vi "Autonomous Independent.vi"() -> ()   [LabVIEW 2016]
doc: "This VI is called when autonomous begins, and will automatically be terminated when autonomous ends. You can carry out timed or sensor driven robot movement independently without needing to return to the caller."
uses:
  <vilib>/Rock Robotics/Network Tables/NT Read Number.vi
  <vilib>/Rock Robotics/WPI/Solenoid/WPI_SolenoidValue.ctl
panel:
  in  "Value":T1=enum."Forward"
  out "Auto Mode":dbl=3.0
  in  "Auton_Modes":T2(array[cluster])=[{"Actions"=[{"Effort"=0.55, "Duration"=3.5, "Action"=enum."Nothing"}, {"Effort"=0.0, "Duration"=0.0, "Action"=enum."Nothing"}]}, {"Actions"=[{"Effort"=0.0, "Duration"=1.0, "Action"=enum."Nothing"}, {"Effort"=0.75, "Duration"=5.0, "Action"=enum."Nothing"}, {"Effort"=0.0, "Duration"=1.0, "Action"=enum."Nothing"}]}, {"Actions"=[{"Effort"=1.0, "Duration"=3.0, "Action"=enum."Nothing"}, {"Effort"=0.0, "Duration"=1.0, "Action"=enum."Nothing"}, {"Effort"=0.75, "Duration"=3.5, "Action"=enum."Nothing"}, {"Effort"=0.0, "Duration"=1.0, "Action"=enum."Nothing"}]}, {"Actions"=[{"Effort"=0.0, "Duration"=0.5, "Action"=enum."Nothing"}, {"Effort"=0.8, "Duration"=5.28, "Action"=enum."Nothing"}, {"Effort"=0.0, "Duration"=1.0, "Action"=enum."Nothing"}, {"Effort"=-0.8, "Duration"=1.8, "Action"=enum."Nothing"}, {"Effort"=0.0, "Duration"=0.1, "Action"=enum."Nothing"}, {"Effort"=0.8, "Duration"=1.75, "Action"=enum."Nothing"}, {"Effort"=0.0, "Duration"=0.5, "Action"=enum."Nothing"}, {"Effort"=0.0, "Duration"=4.0, "Action"=enum."Nothing"}]}, {"Actions"=[{"Effort"=0.0, "Duration"=0.0, "Action"=enum."Nothing"}, {"Effort"=1.0, "Duration"=0.1, "Action"=enum."Nothing"}, {"Effort"=0.0, "Duration"=0.1, "Action"=enum."Nothing"}, {"Effort"=1.0, "Duration"=3.0, "Action"=enum."Nothing"}]}, {"Actions"=[{"Effort"=0.0, "Duration"=0.0, "Action"=enum."Nothing"}, {"Effort"=1.0, "Duration"=0.1, "Action"=enum."Nothing"}, {"Effort"=0.0, "Duration"=0.1, "Action"=enum."Nothing"}, {"Effort"=1.0, "Duration"=3.0, "Action"=enum."Nothing"}]}, {"Actions"=[{"Effort"=0.55, "Duration"=4.0, "Action"=enum."Nothing"}, {"Effort"=0.0, "Duration"=1.0, "Action"=enum."Nothing"}, {"Effort"=-0.5, "Duration"=0.6, "Action"=enum."Nothing"}, {"Effort"=0.75, "Duration"=1.0, "Action"=enum."Nothing"}, {"Effort"=0.0, "Duration"=1.0, "Action"=enum."Nothing"}, {"Effort"=0.75, "Duration"=3.0, "Action"=enum."Nothing"}]}, {"Actions"=[{"Effort"=0.0, "Duration"=0.5, "Action"=enum."Nothing"}, {"Effort"=0.55, "Duration"=4.25, "Action"=enum."Nothing"}, {"Effort"=0.0, "Duration"=0.0, "Action"=enum."Nothing"}, {"Effort"=0.0, "Duration"=0.3, "Action"=enum."Nothing"}, {"Effort"=0.9, "Duration"=2.0, "Action"=enum."Nothing"}]}, {"Actions"=[{"Effort"=0.0, "Duration"=0.0, "Action"=enum."Nothing"}]}]
  # "Nothing"
  # "Boiler Side Gear"
  # "Middle Gear"
  # "Farside Gear"
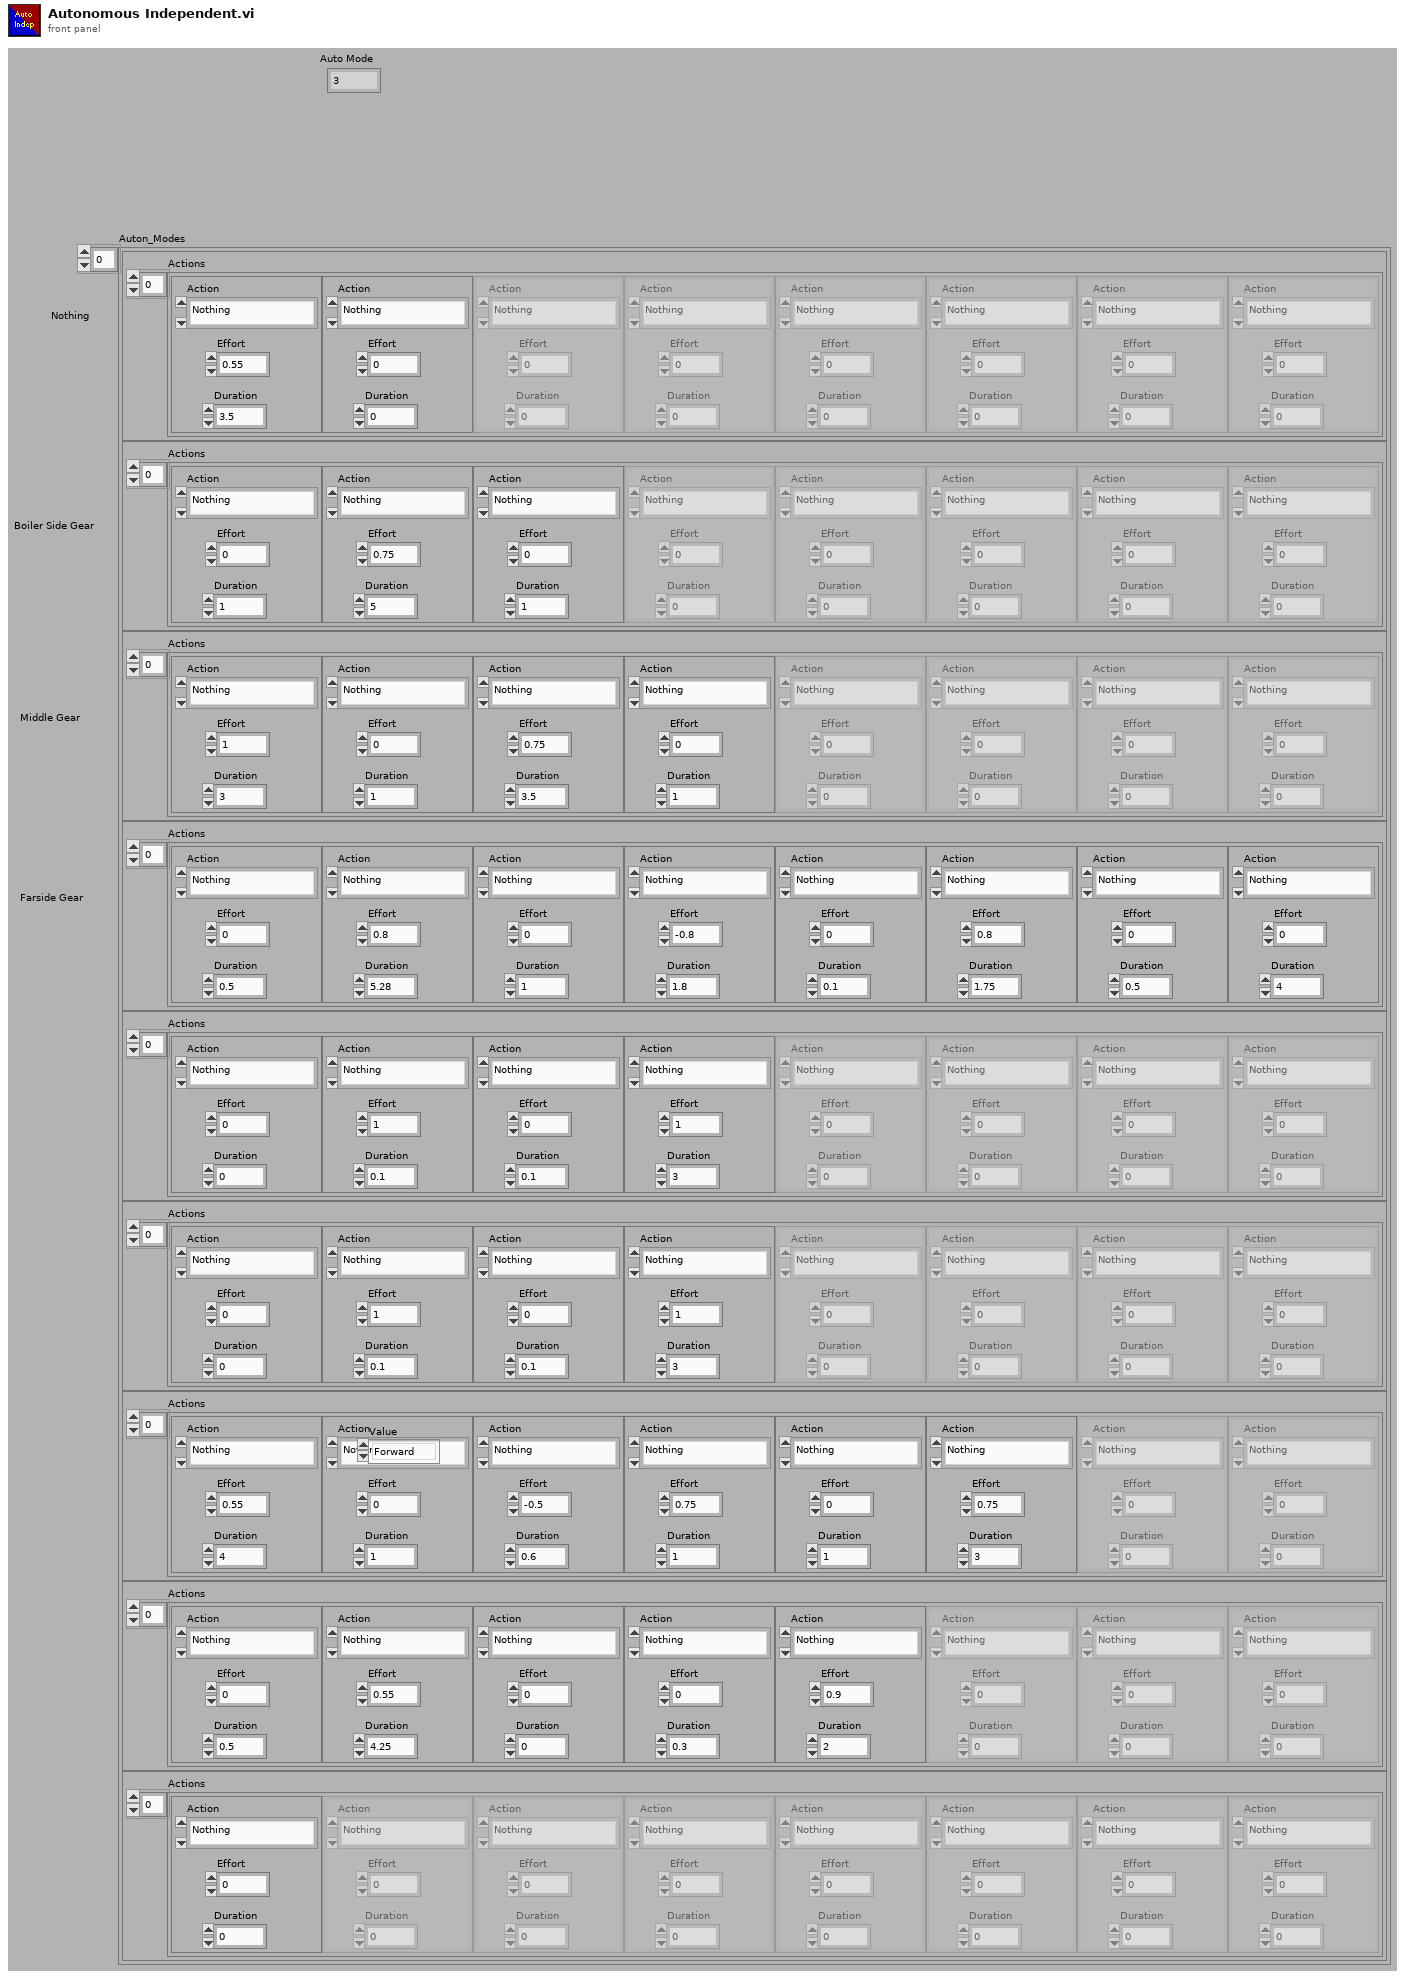
[diagram p1: front panel]
types:
  T1 = typedef "WPI_SolenoidValue.ctl" = enum16{"Off", "On", "Forward", "Reverse"}
  T2 = cluster{"Actions":cluster{"Effort":dbl, "Duration":dbl, "Action":enum16{"Nothing", "Drive", "Turn", "Gear0", "Gear1", "Climb", "Intake", "Index", "Shoot", "Test", "Drive Encoder Reset", "Gyro Reset"}}[]}[]
  T3 = cluster{"Actions":cluster{"Effort":dbl, "Duration":dbl, "Action":enum16{"Nothing", "Drive", "Turn", "Gear0", "Gear1", "Climb", "Intake", "Index", "Shoot", "Test", "Drive Encoder Reset", "Gyro Reset"}}[]}
  T4 = cluster{"Effort":dbl, "Duration":dbl, "Action":enum16{"Nothing", "Drive", "Turn", "Gear0", "Gear1", "Climb", "Intake", "Index", "Shoot", "Test", "Drive Encoder Reset", "Gyro Reset"}}[]
  T5 = enum16{"Nothing", "Drive", "Turn", "Gear0", "Gear1", "Climb", "Intake", "Index", "Shoot", "Test", "Drive Encoder Reset", "Gyro Reset"}
  T6 = typedef "WPI_MotorControlDeviceRef.ctl" = cluster{"DeviceStatus":errorcluster, "Type":T7, "PWM":cluster{"PWM Channel":T8, "DeadBand":T9}, "CAN":cluster{"Device Number":u8, "SetOutput VI Ref":variant, "GetOutput VI Ref":variant, "Enable VI Ref":variant, "Disable VI Ref":variant, "Data":variant}, "Invert":bool}
  T7 = typedef "WPI_MotorControlType.ctl" = enum16{"PWM", "CAN"}
  T8 = typedef "FPGA_DIOPWMChannel.ctl" = enum8{"PWM 0", "PWM 1", "PWM 2", "PWM 3", "PWM 4", "PWM 5", "PWM 6", "PWM 7", "PWM 8", "PWM 9", "PWM MXP 0", "PWM MXP 1", "PWM MXP 2", "PWM MXP 3", "PWM MXP 4", "PWM MXP 5", "PWM MXP 6", "PWM MXP 7", "PWM MXP 8", "PWM MXP 9", "Invalid"}
  T9 = typedef "WPI_PWMDeadband.ctl" = cluster{"Name":string, "maxPositivePwm":i32, "minPositivePwm":i32, "centerPwm":i32, "maxNegativePwm":i32, "minNegativePwm":i32, "angularRange":u16}
  T10 = typedef "WPI_GyroDevRef.ctl" = cluster{"DevStatus":errorcluster, "Analog Channel":T11, "Offset":dbl, "Gain (VoltsPerDegree/Second)":dbl, "Gyro Type":enum16{"Analog", "XRS450"}, "Handle":i32, "SPI Bus":T12, "Device Found":bool, "Sample Rate":dbl, "Calibrate On Open":bool}
  T11 = typedef "FPGA_AIChannel.ctl" = enum8{"AI 0", "AI 1", "AI 2", "AI 3", "AI MXP 0", "AI MXP 1", "AI MXP 2", "AI MXP 3", "Invalid"}
  T12 = typedef "spi_bus.ctl" = enum16{"SPI On-Board, CS0", "SPI On-Board, CS1", "SPI On-Board, CS2", "SPI On-Board, CS3", "SPI MXP", "Invalid"}
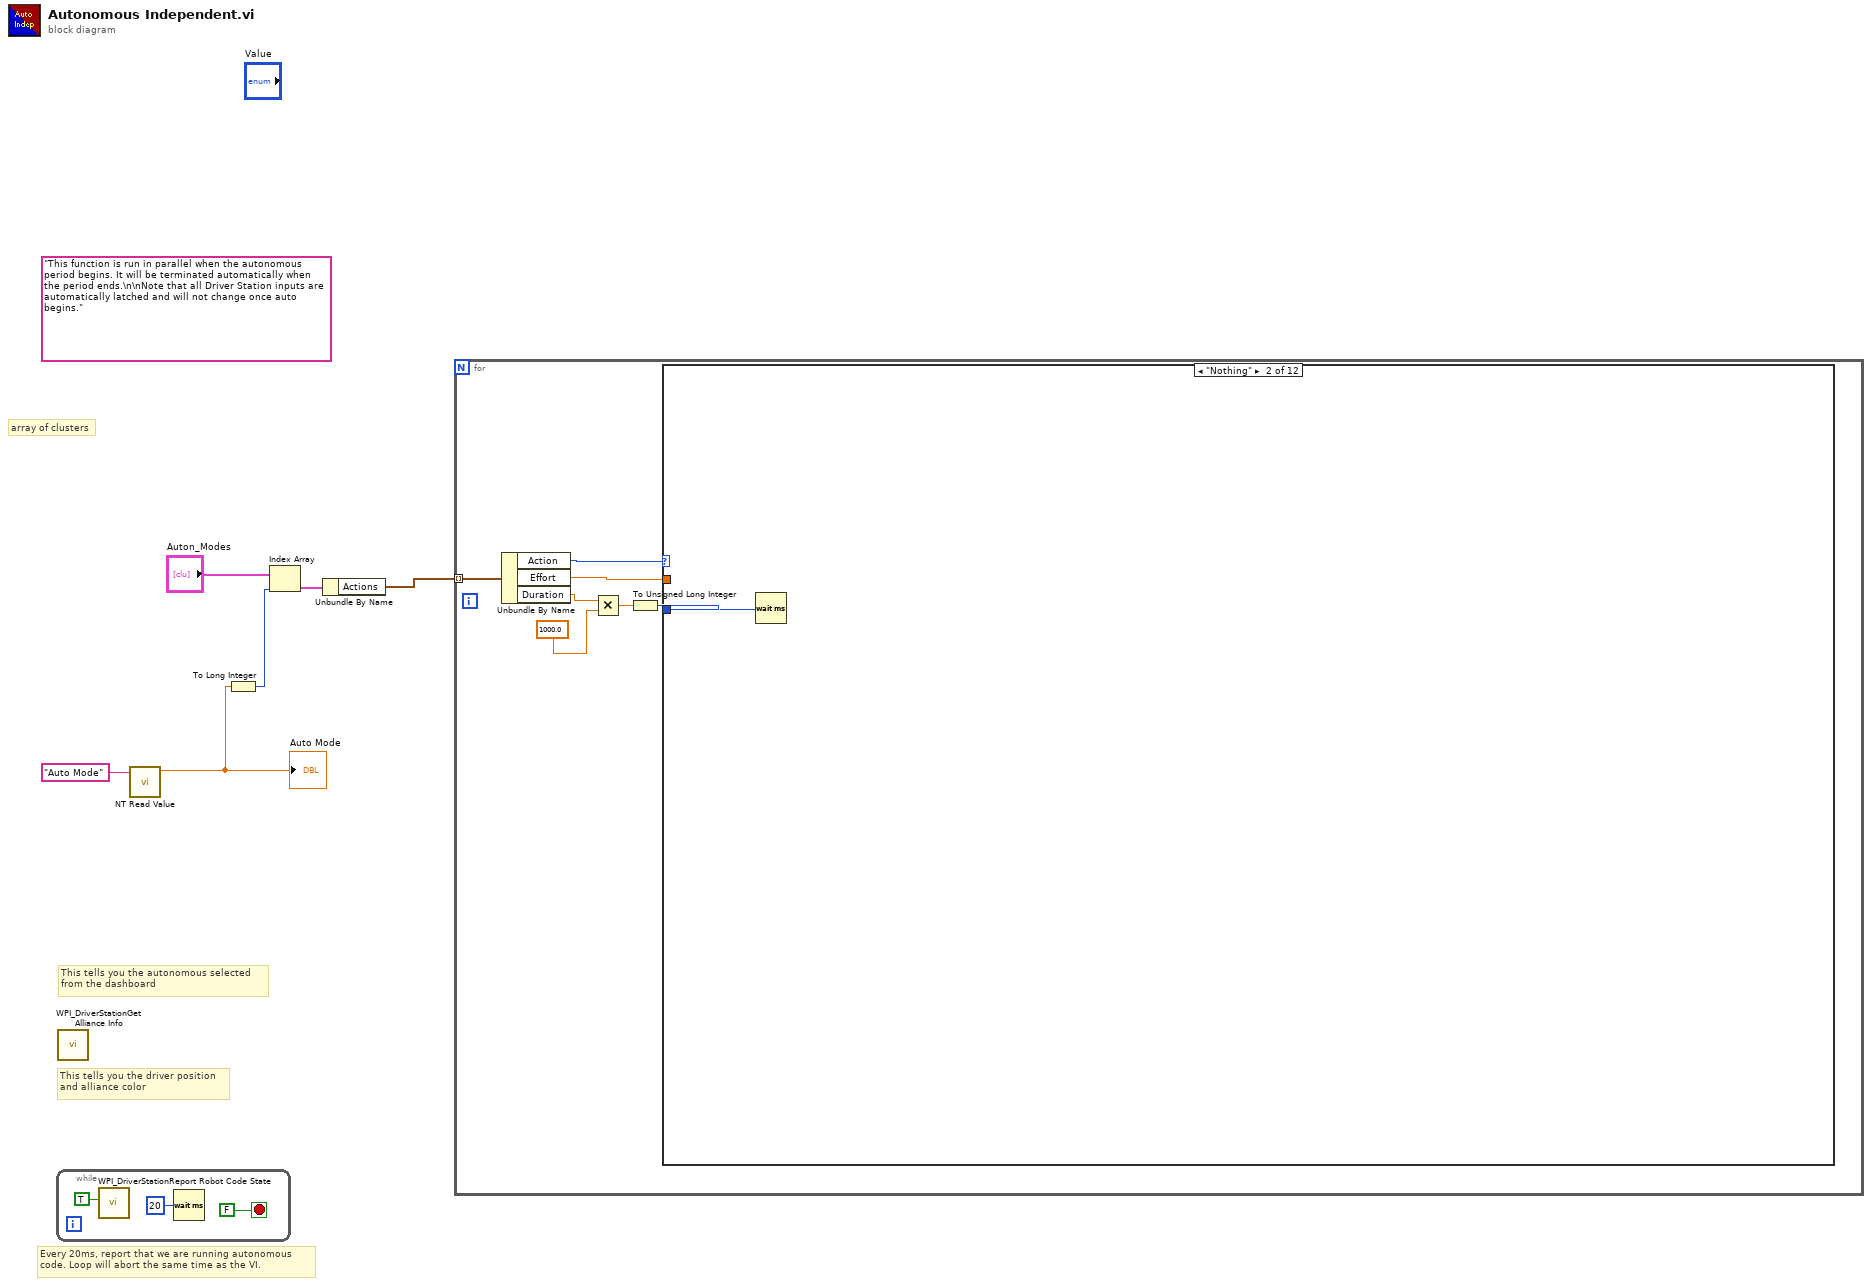
[diagram p0: block diagram]
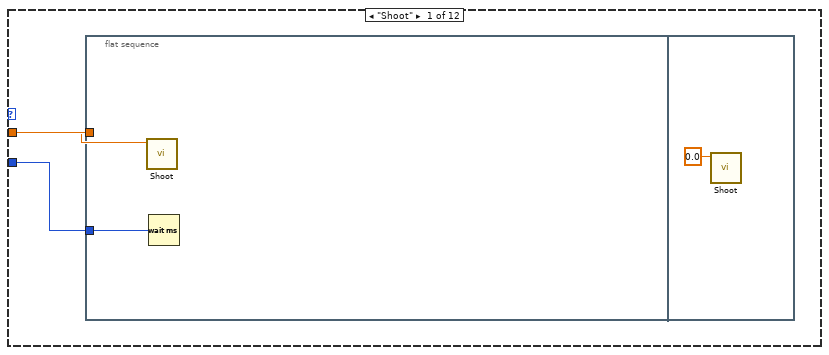
[diagram p2: hidden frame]
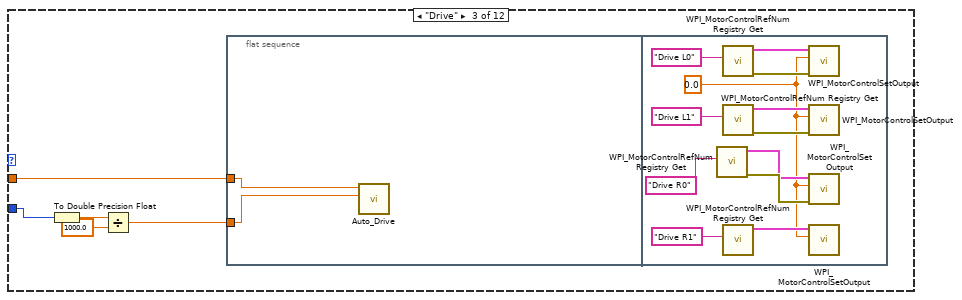
[diagram p3: hidden frame]
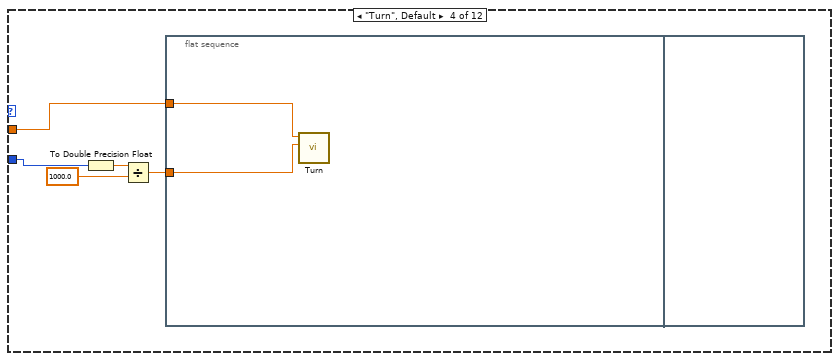
[diagram p4: hidden frame]
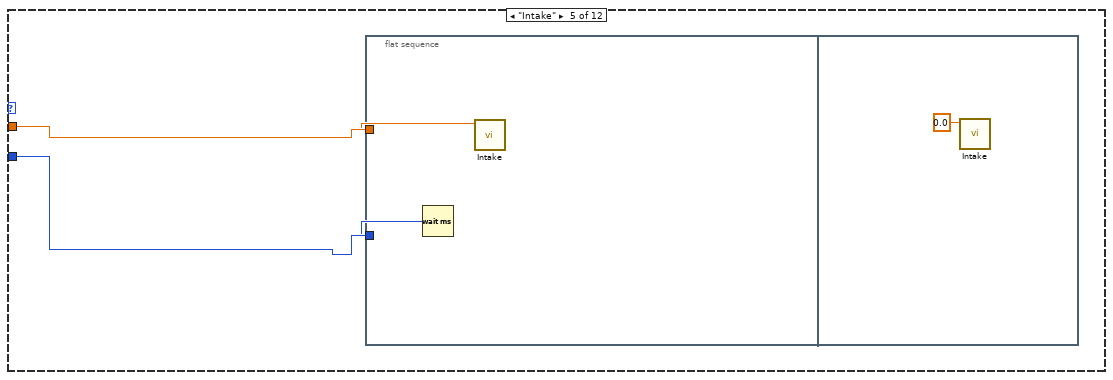
[diagram p5: hidden frame]
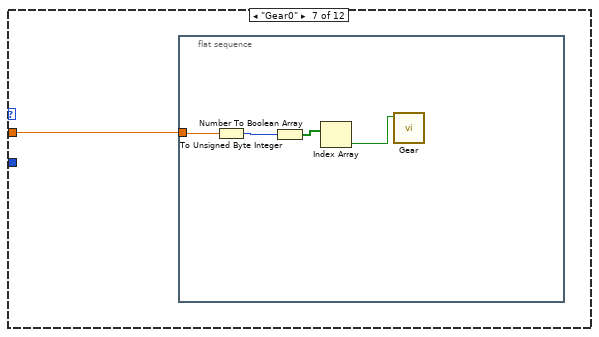
[diagram p7: hidden frame]
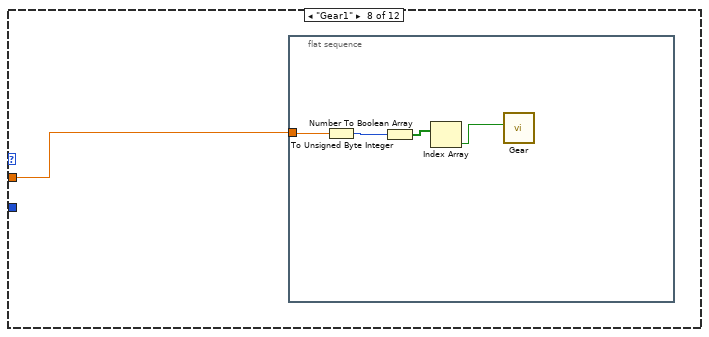
[diagram p8: hidden frame]
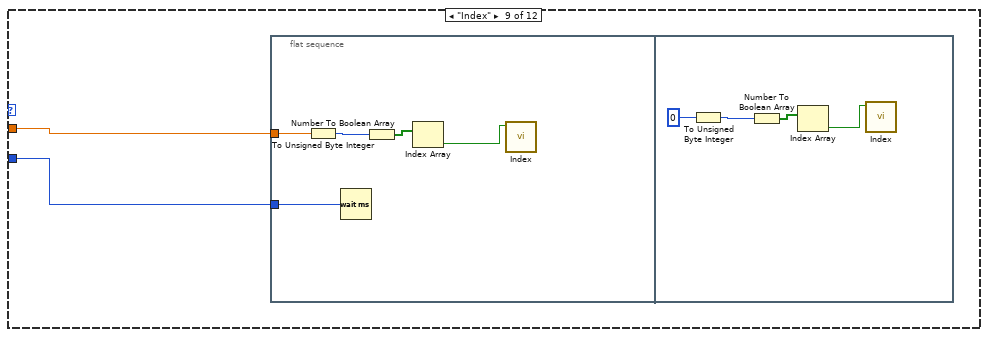
[diagram p9: hidden frame]
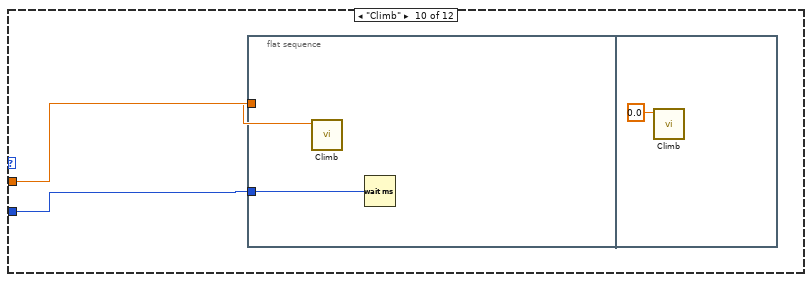
[diagram p10: hidden frame]
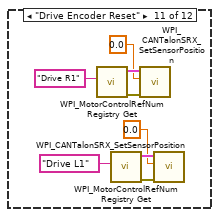
[diagram p11: hidden frame]
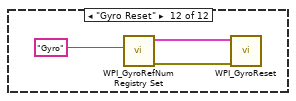
[diagram p12: hidden frame]
diagram:
  (unwired) "This function is run in parallel when the autonomous period begins. It will be terminated automatically when the period ends.\n\nNote that all Driver Station inputs are automatically latched and will not change once auto begins."
  # "This tells you the autonomous selected\nfrom the dashboard"
  # "array of clusters"
  # "Every 20ms, report that we are running autonomous\ncode. Loop will abort the same time as the VI."
  # "This tells you the driver position\nand alliance color"
  n1 = while {
    stop <- FALSE stop-if-true
    n2 = call <vilib>:"WPI_DriverStationReport Robot Code State.vi"("Autonomous"=TRUE) -> ()  [unwired: 10 in, 1 out]
    n3 = Wait (ms)(milliseconds to wait=u32 20) -> ()  [unwired: 1 out]
  }
  n4 = call <vilib>:"WPI_DriverStationGet Alliance Info.vi"() -> ()  [unwired: 12 out]
  n5 = call-poly <vilib>:"NT Read Value.vi"("Name"="Auto Mode") -> ("Numeric"=w1:dbl)  [unwired: 9 in, 1 out]
  "Auto Mode" <- w1
  n6 = To Long Integer(number=w1) -> (32bit integer=w3:i32)
  n7 = Index Array(array="Auton_Modes", index=w3) -> (element=w5:T3)
  n8 = Unbundle By Name(w5) -> ("Actions"=w6:T4)
  n9 = for {
    tunnel: w6 -> [w16] mode=indexing
    n10 = Unbundle By Name(w16) -> ("Action"=w15:T5, "Effort"=w14:dbl, "Duration"=w13:dbl)
    n11 = Multiply(x=w13, y=1000.0) -> (x*y=w11:dbl)
    n12 = To Unsigned Long Integer(number=w11) -> (unsigned 32bit integer=w10:u32)
    n13 = case shown="\"Nothing\"" w15 {
      tunnel: w14 -> [w18 _ w27 w46 w50 _ w54 w59 w64 w76 _ _]
      tunnel: w10 -> [w17 w22 w26 w45 w49 _ _ _ w65 w75 _ _]
      frame "Shoot" {
        n14 = flat-sequence {
          tunnel: w18 -> [w20]
          tunnel: w17 -> [w19]
          frame #0 {
            n15 = call "Shoot.vi"("Effort"=w20) -> ()  [unwired: 11 in]
            n16 = Wait (ms)(milliseconds to wait=w19) -> ()  [unwired: 1 out]
          }
          frame #1 {
            n17 = call "Shoot.vi"("Effort"=0.0) -> ()  [unwired: 11 in]
          }
        }
      }
      frame "Nothing" {
        n18 = Wait (ms)(milliseconds to wait=w22) -> ()  [unwired: 1 out]
      }
      frame "Drive" {
        n19 = To Double Precision Float(number=w26) -> (double precision float=w25:dbl)
        n20 = Divide(x=w25, y=1000.0) -> (x/y=w23:dbl)
        n21 = flat-sequence {
          tunnel: w27 -> [w29]
          tunnel: w23 -> [w28]
          frame #0 {
            n22 = call "Auto_Drive.vi"("Duration"=w28, "Drive Effort"=w29) -> ()  [unwired: 10 in]
          }
          frame #1 {
            w30 = 0.0 ("Drive L")
            n23 = call <vilib>:"WPI_MotorControlRefNum Registry Get.vi"("refnum name"="Drive R0") -> ("error out"=w35:errorcluster, "MotorControlDevRef"=w31:T6)  [unwired: 9 in]
            n24 = call <vilib>:"WPI_MotorControlRefNum Registry Get.vi"("refnum name"="Drive L0") -> ("error out"=w36:errorcluster, "MotorControlDevRef"=w37:T6)  [unwired: 9 in]
            n25 = call <vilib>:"WPI_MotorControlRefNum Registry Get.vi"("refnum name"="Drive L1") -> ("error out"=w40:errorcluster, "MotorControlDevRef"=w39:T6)  [unwired: 9 in]
            n26 = call <vilib>:"WPI_MotorControlRefNum Registry Get.vi"("refnum name"="Drive R1") -> ("MotorControlDevRef"=w33:T6)  [unwired: 9 in, 1 out]
            n27 = call <vilib>:"WPI_MotorControlSetOutput.vi"("error in (no error)"=w36, "Output"=w30, "MotorControlDevRef"=w37) -> ()  [unwired: 6 in, 3 out]
            n28 = call <vilib>:"WPI_MotorControlSetOutput.vi"("error in (no error)"=w40, "Output"=w30, "MotorControlDevRef"=w39) -> ()  [unwired: 6 in, 3 out]
            n29 = call <vilib>:"WPI_MotorControlSetOutput.vi"("error in (no error)"=w35, "Output"=w30, "MotorControlDevRef"=w31) -> ()  [unwired: 6 in, 3 out]
            n30 = call <vilib>:"WPI_MotorControlSetOutput.vi"("Output"=w30, "MotorControlDevRef"=w33) -> ()  [unwired: 7 in, 3 out]
          }
        }
      }
      frame "Turn", Default {
        n31 = To Double Precision Float(number=w45) -> (double precision float=w44:dbl)
        n32 = Divide(x=w44, y=1000.0) -> (x/y=w42:dbl)
        n33 = flat-sequence {
          tunnel: w46 -> [w48]
          tunnel: w42 -> [w47]
          frame #0 {
            n34 = call "Turn.vi"("Angle"=w47, "Effort"=w48) -> ()  [unwired: 10 in]
          }
          frame #1 {
          }
        }
      }
      frame "Intake" {
        n35 = flat-sequence {
          tunnel: w50 -> [w52]
          tunnel: w49 -> [w51]
          frame #0 {
            n36 = Wait (ms)(milliseconds to wait=w51) -> ()  [unwired: 1 out]
            n37 = call "Intake.vi"("Effort"=w52) -> ()  [unwired: 11 in]
          }
          frame #1 {
            n38 = call "Intake.vi"("Effort"=0.0) -> ()  [unwired: 11 in]
          }
        }
      }
      frame "Test" {
      }
      frame "Gear0" {
        n39 = flat-sequence {
          tunnel: w54 -> [w58]
          frame #0 {
            n40 = To Unsigned Byte Integer(number=w58) -> (unsigned 8bit integer=w57:u8)
            n41 = Number To Boolean Array(number=w57) -> (Boolean array=w56:bool[])
            n42 = Index Array(array=w56) -> (element=w55:bool)  [unwired: 1 in]
            n43 = call "Gear.vi"("Gear0?"=w55) -> ()  [unwired: 11 in]
          }
        }
      }
      frame "Gear1" {
        n44 = flat-sequence {
          tunnel: w59 -> [w63]
          frame #0 {
            n45 = To Unsigned Byte Integer(number=w63) -> (unsigned 8bit integer=w62:u8)
            n46 = Number To Boolean Array(number=w62) -> (Boolean array=w61:bool[])
            n47 = Index Array(array=w61) -> (element=w60:bool)  [unwired: 1 in]
            n48 = call "Gear.vi"("Gear1?"=w60) -> ()  [unwired: 11 in]
          }
        }
      }
      frame "Index" {
        n49 = flat-sequence {
          tunnel: w65 -> [w67]
          tunnel: w64 -> [w66]
          frame #0 {
            n50 = To Unsigned Byte Integer(number=w66) -> (unsigned 8bit integer=w70:u8)
            n51 = Wait (ms)(milliseconds to wait=w67) -> ()  [unwired: 1 out]
            n52 = Number To Boolean Array(number=w70) -> (Boolean array=w69:bool[])
            n53 = Index Array(array=w69) -> (element=w68:bool)  [unwired: 1 in]
            n54 = call "Index.vi"("Index?"=w68) -> ()  [unwired: 11 in]
          }
          frame #1 {
            n55 = To Unsigned Byte Integer(number=u8 0) -> (unsigned 8bit integer=w73:u8)
            n56 = Number To Boolean Array(number=w73) -> (Boolean array=w74:bool[])
            n57 = Index Array(array=w74) -> (element=w71:bool)  [unwired: 1 in]
            n58 = call "Index.vi"("Index?"=w71) -> ()  [unwired: 11 in]
          }
        }
      }
      frame "Climb" {
        n59 = flat-sequence {
          tunnel: w76 -> [w78]
          tunnel: w75 -> [w77]
          frame #0 {
            n60 = call "Climb.vi"("Effort"=w78) -> ()  [unwired: 11 in]
            n61 = Wait (ms)(milliseconds to wait=w77) -> ()  [unwired: 1 out]
          }
          frame #1 {
            n62 = call "Climb.vi"("Effort"=0.0) -> ()  [unwired: 11 in]
          }
        }
      }
      frame "Drive Encoder Reset" {
        n63 = call <vilib>:"WPI_MotorControlRefNum Registry Get.vi"("refnum name"="Drive R1") -> ("error out"=w82:errorcluster, "MotorControlDevRef"=w81:T6)  [unwired: 9 in]
        n64 = call <vilib>:"WPI_MotorControlRefNum Registry Get.vi"("refnum name"="Drive L1") -> ("error out"=w84:errorcluster, "MotorControlDevRef"=w85:T6)  [unwired: 9 in]
        n65 = call <vilib>:"WPI_CANTalonSRX_SetSensorPosition.vi"("error in (no error)"=w82, "New Sensor Position"=0.0, "CAN Talon SRX Ref"=w81) -> ()  [unwired: 7 in, 2 out]
        n66 = call <vilib>:"WPI_CANTalonSRX_SetSensorPosition.vi"("error in (no error)"=w84, "New Sensor Position"=0.0, "CAN Talon SRX Ref"=w85) -> ()  [unwired: 7 in, 2 out]
      }
      frame "Gyro Reset" {
        n67 = call <vilib>:"WPI_GyroRefNum Registry Set.vi"("refnum name"="Gyro") -> ("error out"=w89:errorcluster, "GyroDevRef"=w90:T10)  [unwired: 9 in]
        n68 = call <vilib>:"WPI_GyroReset.vi"("error in"=w89, "GyroDevRef"=w90) -> ()  [unwired: 8 in, 2 out]
      }
    }
  }
